vi "Get Main VI Refs.vi"(8 "error in":errorcluster, 11 "Project":refnum<class "Project.lvclass">) -> (0 "error out":errorcluster, 3 "HL Cluster":T1, 5 "Refresh Time":i32)   [LabVIEW 2020, in "Panther Dashboard.lvlib"]
uses:
  Panther Dashboard.lvlib
  Class/Project/Project.lvclass
  C:/GitClones/PantherDashboard/src/LabVIEW/Panther Dashboard/Class/LabVIEWItem/LabVIEWItem.lvclass
  Helper Loop--cluster.ctl
  Module type--enum.ctl
  Class/Project/Project.lvclass/Project.ctl
  Class/LabVIEWItem/LabVIEWItem.lvclass/LabVIEWItem.ctl
  Class/Library/Library.lvclass/Library.ctl
  Class/LabVIEWItem/Read Item Path.vi
  Class/LabVIEWItem/Read Item Name.vi
  Class/Library/Read Type.vi
  Class/Library/Read Dependency.vi
  Class/Library/Get HSE module.vi
  Class/Project/Read Libraries.vi
  Class/Project/Read Target App Ins Ref.vi
  Class/Project/Read Target Name.vi
  Class/Library/Library.lvclass
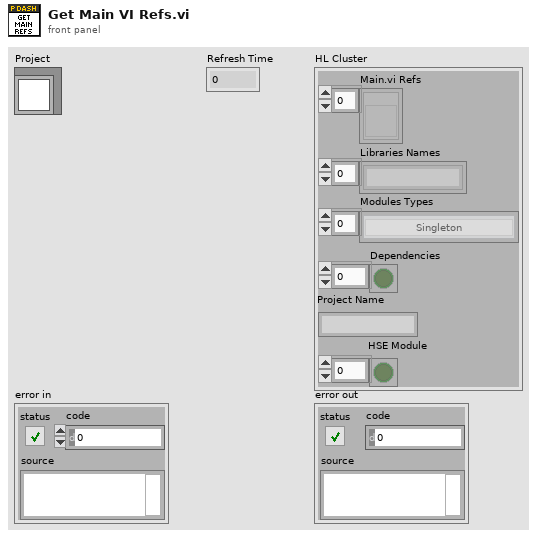
[diagram p1: front panel]
types:
  T1 = typedef "Panther Dashboard.lvlib/Helper Loop--cluster.ctl" = cluster{"Main.vi Refs":refnum<vi>[], "Libraries Names":string[], "Modules Types":T2[], "Dependencies":bool[], "Project Name":string, "HSE Module":bool[]}
  T2 = typedef "Panther Dashboard.lvlib/Module type--enum.ctl" = enum16{"Singleton", "Cloneable"}
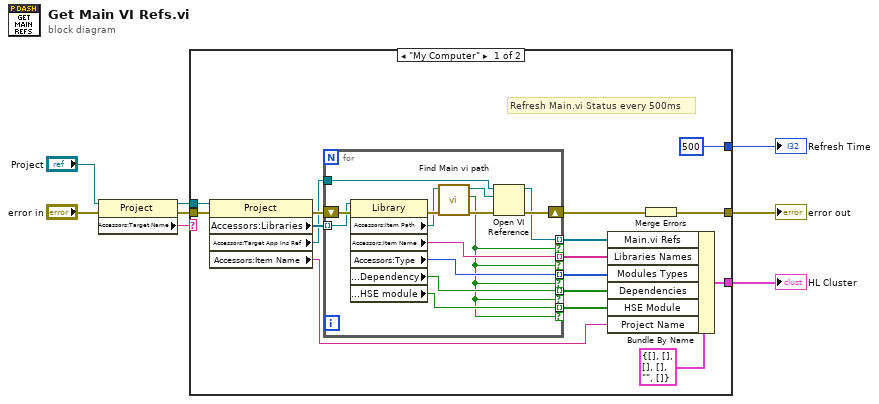
[diagram p0: block diagram]
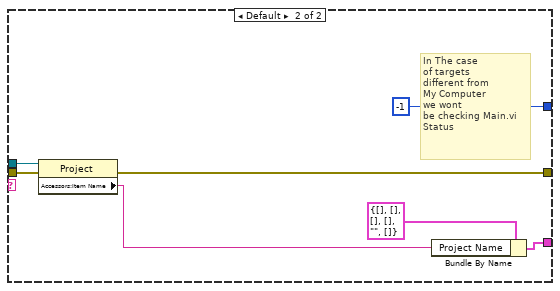
[diagram p2: hidden frame]
diagram:
  n1 = property class="Project"(reference="Project", error in="error in") -> (reference out=w2:refnum<class "Project.lvclass">, error out=w6:errorcluster, "Accessors:Target Name"=w1:string)
  n2 = case shown="\"My Computer\"" w1 {
    tunnel: [w24 w45] -> w8
    tunnel: w6 -> [w22 w44]
    tunnel: w2 -> [w20 w43]
    tunnel: [w16 w41] -> w5
    tunnel: [500 -1] -> w4
    frame "My Computer" {
      # "Refresh Main.vi Status every 500ms"
      n3 = property class="Project"(reference=w20, error in=w22) -> (error out=w23:errorcluster, "Accessors:Libraries"=w19:refnum<class "Library.lvclass">[], "Accessors:Target App Ins Ref"=w18:refnum<vi>, "Accessors:Item Name"=w12:string)  [unwired: 1 out]
      n4 = for {
        tunnel: [w34] -> w15 mode=indexing if=w25
        tunnel: w19 -> [w33] mode=indexing
        tunnel: w18 -> [w27]
        tunnel: [w32] -> w14 mode=indexing if=w25
        tunnel: [w31] -> w13 mode=indexing if=w25
        shift-right: [w35] -> w21
        shift-left: w23 -> [w37]
        tunnel: [w28] -> w10 mode=indexing if=w25
        tunnel: [w26] -> w9 mode=indexing if=w25
        n5 = property class="Library"(reference=w33, error in=w37) -> (error out=w38:errorcluster, "Accessors:Item Path"=w30:path, "Accessors:Item Name"=w34:string, "Accessors:Type"=w32:T2, "Accessors:Dependency"=w31:bool, "Accessors:HSE module"=w26:bool)  [unwired: 1 out]
        n6 = call "Find Main vi path.vi"("error in"=w38, "Library Path"=w30) -> ("error out"=w36:errorcluster, "Main.vi Found?"=w25:bool, "Main vi Path"=w29:path)  [unwired: 7 in]
        n7 = Open VI Reference(application reference (local)=w27, vi path=w29, error in (no error)=w36) -> (vi reference=w28:refnum<vi>, error out=w35:errorcluster)  [unwired: 3 in]
      }
      n8 = Bundle By Name(cluster=T1 {"Main.vi Refs"=[], "Libraries Names"=[], "Modules Types"=[], "Dependencies"=[], "Project Name"="", "HSE Module"=[]} ("Helper Loop Cluster"), "Main.vi Refs"=w10, "Libraries Names"=w15, "Modules Types"=w14, "Dependencies"=w13, "HSE Module"=w9, "Project Name"=w12) -> (w16:T1)
      n9 = Merge Errors(w21) -> (w24:errorcluster)
    }
    frame Default {
      # "In The case\nof targets\ndifferent from\nMy Computer\nwe wont\nbe checking Main.vi\nStatus"
      n10 = property class="Project"(reference=w43, error in=w44) -> (error out=w45:errorcluster, "Accessors:Item Name"=w40:string)  [unwired: 1 out]
      n11 = Bundle By Name(cluster=T1 {"Main.vi Refs"=[], "Libraries Names"=[], "Modules Types"=[], "Dependencies"=[], "Project Name"="", "HSE Module"=[]} ("Helper Loop Cluster"), "Project Name"=w40) -> (w41:T1)
    }
  }
  "error out" <- w8
  "HL Cluster" <- w5
  "Refresh Time" <- w4
